vi "fgv_measure_rc.vi"(7 "cmd":T2, 11 "measure_rc":T1) -> (3 "measure_rc 2":T1 {"전압강하" format="%.3f"; "충전전압 63초" format="%.3f"})   [LabVIEW 2019]
uses:
  measure_rc.ctl
  _ctrl/rw.ctl
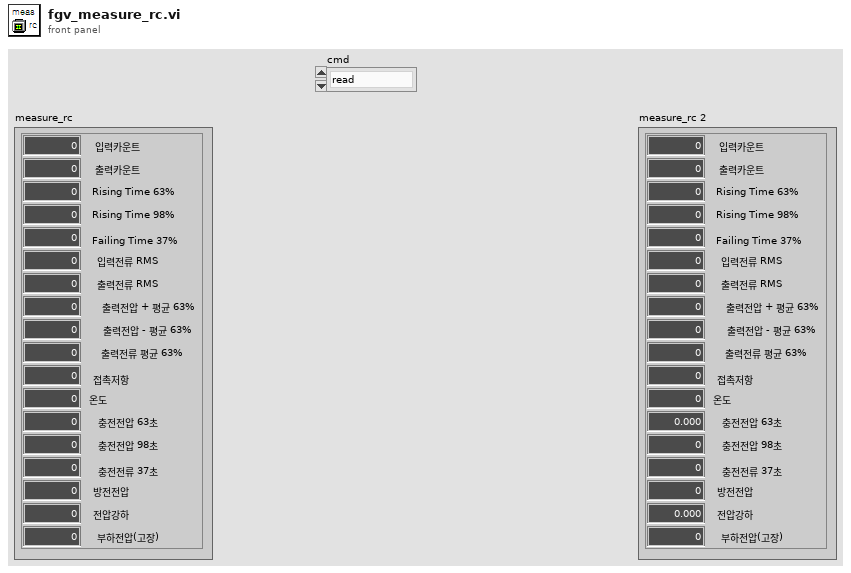
[diagram p1: front panel]
types:
  T1 = typedef "measure_rc.ctl" = cluster{"입력카운트":dbl, "출력카운트":dbl, "Rising Time 63%":dbl, "Rising Time 98%":dbl, "Failing Time 37%":dbl, "입력전류 RMS":dbl, "출력전류 RMS":dbl, "출력전압 + 평균 63%":dbl, "출력전압 - 평균 63%":dbl, "출력전류 평균 63%":dbl, "접촉저항":dbl, "온도":dbl, "충전전압 63초":dbl, "충전전압 98초":dbl, "충전전류 37초":dbl, "방전전압":dbl, "전압강하":dbl, "부하전압(고장)":dbl}
  T2 = typedef "rw.ctl" = enum16{"read", "write"}
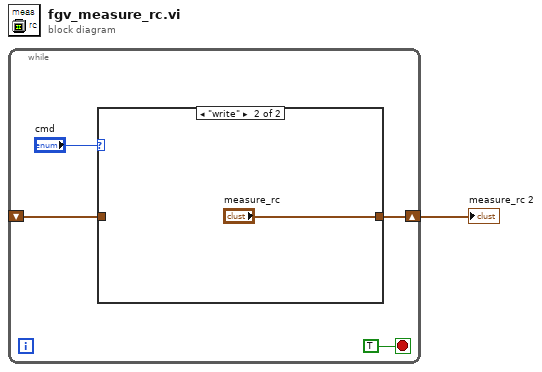
[diagram p0: block diagram]
diagram:
  n1 = while {
    shift-right: [w3] -> w1
    shift-left: _ -> [w2]
    stop <- TRUE stop-if-true
    n2 = case shown="\"write\"" "cmd" {
      tunnel: [w6 "measure_rc"] -> w3
      tunnel: w2 -> [w6 _]
      frame "read", Default {
      }
      frame "write" {
      }
    }
  }
  "measure_rc 2" <- w1
